vi "Read CMD.vi"(8 "error in (no error)":errorcluster, 11 "ePAS in":refnum<class "ePAS.lvclass">) -> (0 "error out":errorcluster, 2 "CMD":refnum<queue>, 3 "ePAS out":refnum<class "ePAS.lvclass">)   [LabVIEW 2014, in "PAS Actor Lib.lvlib" / "ePAS.lvclass"]
uses:
  ePAS.lvclass
  reusable/Command/Command.lvclass
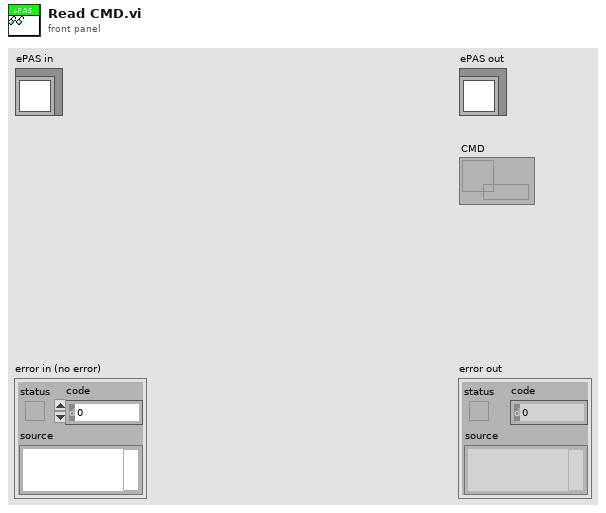
[diagram p1: front panel]
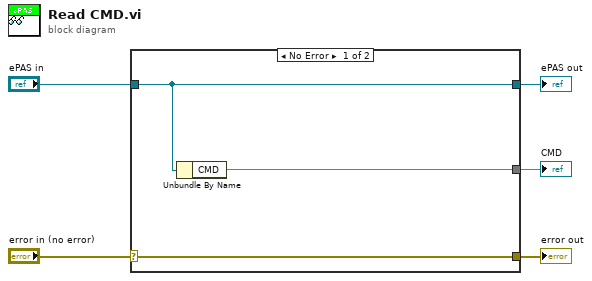
[diagram p0: block diagram]
diagram:
  n1 = case shown="No Error" "error in (no error)" {
    selector: "error in (no error)" -> [w8 w9]
    tunnel: [w8 w9] -> w4
    tunnel: [w7 w10] -> w2
    tunnel: "ePAS in" -> [w7 w10]
    tunnel: [w6 _] -> w1
    frame No Error {
      n2 = Unbundle By Name(w7) -> ("CMD"=w6)
    }
    frame Error {
    }
  }
  "error out" <- w4
  "ePAS out" <- w2
  "CMD" <- w1
